vi "Trim Elf Claims.vi"(8 "error in (no error)":errorcluster, 11 "1D String Array":string[](array[string])) -> (0 "error out":errorcluster, 3 "Trimmed Array":string[](array[string]))   [LabVIEW 2019]
doc: "Trim strings that look like #1 @ 265,241: 16x26 so that they look like 265,241,16,26."
uses:
  <vilib>/regexp/Match Regular Expression.xnode
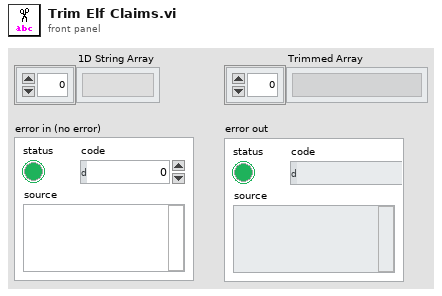
[diagram p1: front panel]
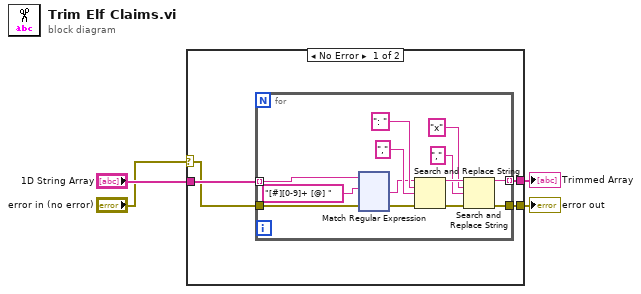
[diagram p0: block diagram]
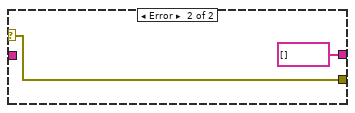
[diagram p2: hidden frame]
diagram:
  n1 = case shown="No Error" "error in (no error)" {
    selector: "error in (no error)" -> [w5 w137]
    tunnel: [w8 string[] []] -> w4
    tunnel: [w7 w137] -> w3
    tunnel: "1D String Array" -> [w6 _]
    frame No Error {
      n2 = for {
        tunnel: w6 -> [w13] mode=indexing
        tunnel: w5 -> [w11]
        tunnel: [w15] -> w8 mode=indexing
        tunnel: [w14] -> w7
        n3 = xnode "Match Regular Expression"("input string"=w13, "regular expression"="[#][0-9]+ [@] " ("search string"), "error in"=w11) -> ("after match"=w9:string, "error out"=w10:errorcluster)  [unwired: 3 in, 3 out]
        n4 = Search and Replace String(input string=w9, search string=": ", replace string="," ("replace string (\"\")"), error in=w10) -> (result string=w19:string, error out=w18:errorcluster)  [unwired: 4 in, 2 out]
        n5 = Search and Replace String(input string=w19, search string="x", replace string="," ("replace string (\"\")"), error in=w18) -> (result string=w15:string, error out=w14:errorcluster)  [unwired: 4 in, 2 out]
      }
    }
    frame Error {
    }
  }
  "error out" <- w3
  "Trimmed Array" <- w4
